vi "GetType.vi"(8 "error in (no error)":errorcluster, 11 "Send Software Stop Trigger [SPT] Msg in":refnum<class "Send Software Stop Trigger [SPT] Msg.lvclass">) -> (0 "error out":errorcluster, 2 "Data Sample":variant, 3 "Send Software Stop Trigger [SPT] Msg out":refnum<class "Send Software Stop Trigger [SPT] Msg.lvclass">)   [LabVIEW 2014, in "CS++Fgen.lvlib" / "Send Software Stop Trigger [SPT] Msg.lvclass"]
doc: "This VI delivers a sample of the data type format the message expects."
uses:
  Send Software Stop Trigger [SPT] Msg.lvclass
  Send Software Stop Trigger [SPT] Msg.lvclass/Send Software Stop Trigger [SPT] Msg.ctl
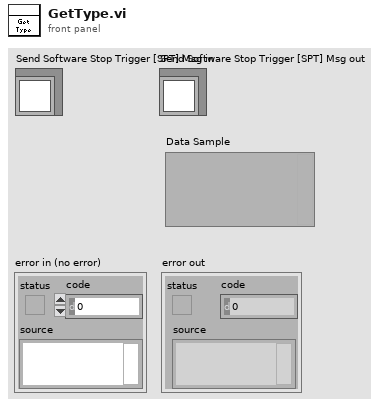
[diagram p1: front panel]
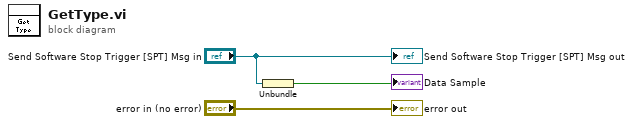
[diagram p0: block diagram]
diagram:
  n1 = Unbundle("Send Software Stop Trigger [SPT] Msg in") -> (→"Data Sample":bool)
  "error out" <- "error in (no error)"
  "Send Software Stop Trigger [SPT] Msg out" <- "Send Software Stop Trigger [SPT] Msg in"
